vi "Database.GetAllStatus.vi"(8 "error in":errorcluster, 9 "Serial":string, 10 "Variant":string, 11 "Data in":T1) -> (0 "error out":errorcluster, 3 "Data out":T1)   [LabVIEW 2016]
uses:
  Database.Data.ctl
  Database.Data.Sets.ctl
  Handler/Database.Handler.Data.Status.ctl
  Database.Gui.ctl
  Database.Gui.SingleTestValue.ctl
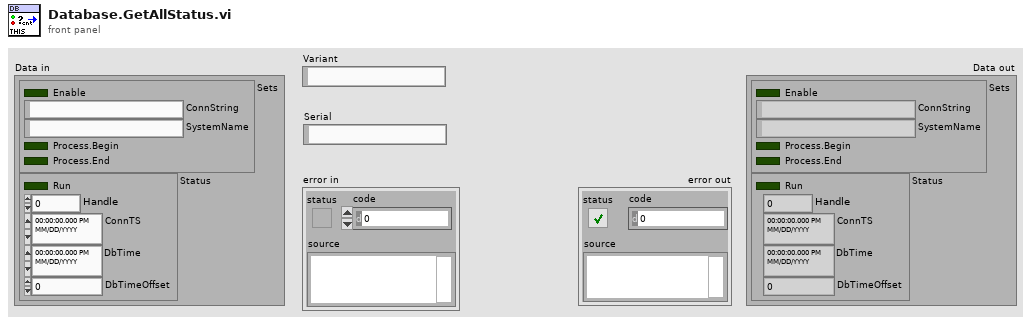
[diagram p1: front panel]
types:
  T1 = typedef "Database.Data.ctl" = cluster{"Sets":T2, "Status":T3}
  T2 = typedef "Database.Data.Sets.ctl" = cluster{"Enable":bool, "ConnString":string, "SystemName":string, "Process.Begin":bool, "Process.End":bool}
  T3 = typedef "Database.Handler.Data.Status.ctl" = cluster{"Run":bool, "Handle":i32, "ConnTS":timestamp, "DbTime":timestamp, "DbTimeOffset":dbl}
  T4 = typedef "Database.Gui.SingleTestValue.ctl" = cluster{"EV_name":string, "Value":dbl, "LimitL":dbl, "LimitH":dbl, "Status":u8}
  T5 = typedef "Database.Gui.ctl" = cluster{"Station":string, "ButtonEnabled":bool, "Values":T4[]}
  T6 = typedef "ProdaNG.Identification.ctl" = cluster{"processId":i32, "systemId":i32, "processStepId":i32, "wabcoPartId":i32}
  T7 = typedef "ProdaNG.Product.ctl" = cluster{"c_id":string, "wabcoPartId":i32, "serialNumber":string, "comment":string, "individual":i32, "crProcessStepId":i32, "mdProcessStepId":i32, "crTime":string, "mdTime":string}
  T8 = typedef "ProdaNG.TestStep.ctl" = cluster{"i_id":i32, "processStepId":i32, "testSequence":i32, "testOrder":i32, "mdReason":string, "mdUser":string, "mdTime":string, "description":string}
  T9 = typedef "ProdaNG.TestValue.ctl" = cluster{"i_id":i32, "testStepId":i32, "releaseId":i32, "unitId":i32, "contentId":string, "previewId":string, "maximum":dbl, "minimum":dbl, "valueText":string, "testValueSequence":i32, "history":i32, "mdReason":string, "mdUser":string, "mdTime":string, "description":string}
  T10 = typedef "ProdaNG.ProcessResult.ctl" = cluster{"c_id":string, "productId":string, "processId":i32, "statusId":i32, "startTime":string, "endTime":string}
  T11 = typedef "ProdaNG.ProcessStepResult.ctl" = cluster{"c_id":string, "processResultId":string, "processStepId":i32, "statusId":i32, "operatorId":i32, "startTime":string, "endTime":string}
  T12 = typedef "ProdaNG.TestStepResult.ctl" = cluster{"c_id":string, "processStepResultId":string, "testStepId":i32, "statusId":i32}
  T13 = typedef "ProdaNG.TestValueResult.ctl" = cluster{"c_id":string, "testStepResultId":string, "testValueId":i32, "result":dbl, "statusId":i32, "contentId":string}
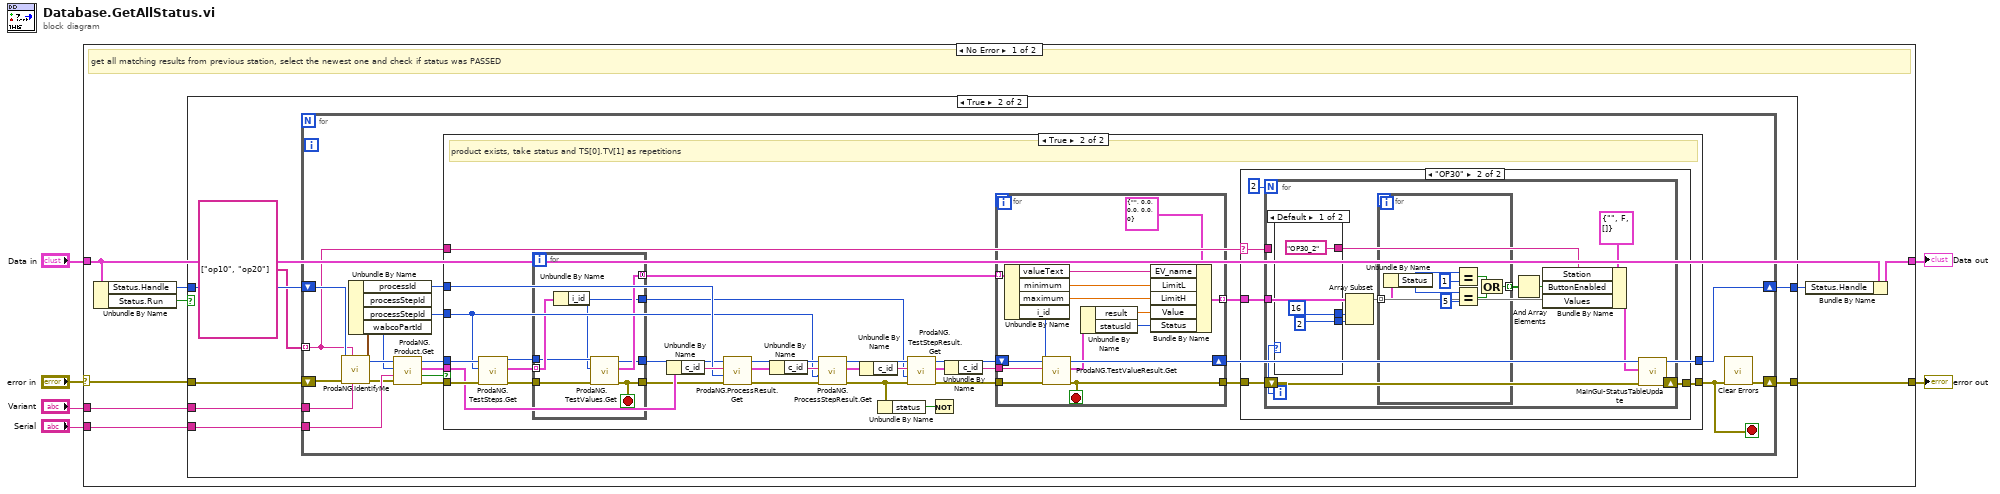
[diagram p0: block diagram]
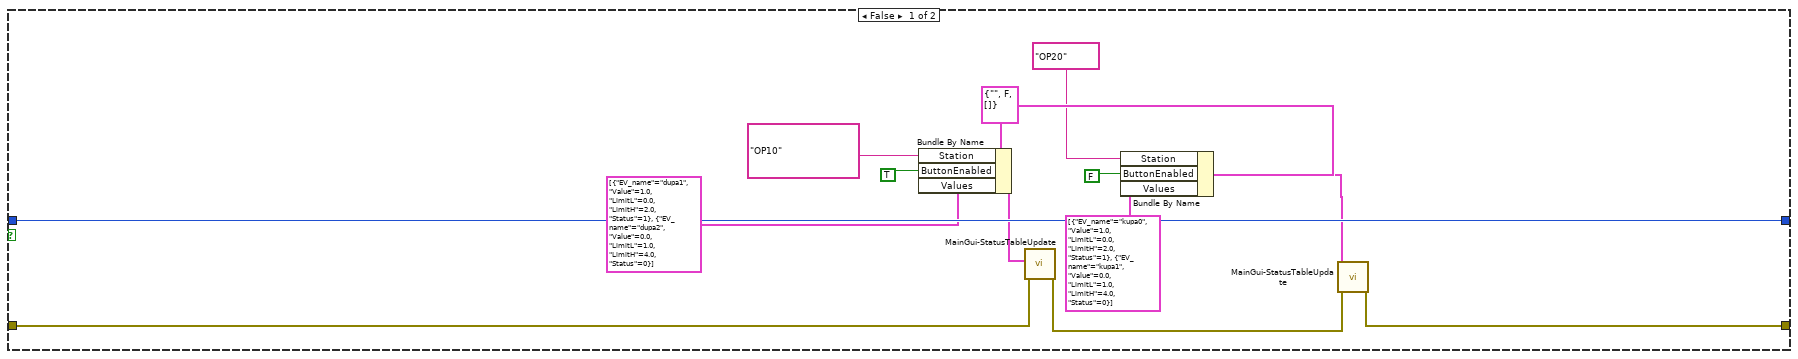
[diagram p2: hidden frame]
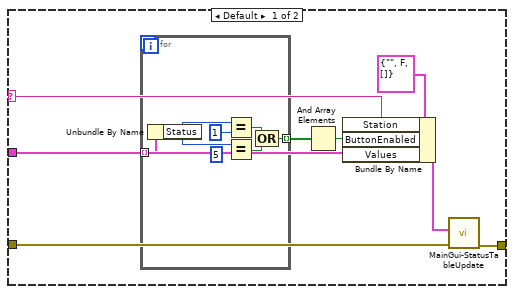
[diagram p4: hidden frame]
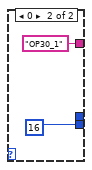
[diagram p5: hidden frame]
diagram:
  n1 = case shown="No Error" "error in" {
    selector: "error in" -> [w14 w154]
    tunnel: [w15 w154] -> w6
    tunnel: "Data in" -> [w12 w153]
    tunnel: [w11 w153] -> w3
    tunnel: "Serial" -> [w8 _]
    tunnel: "Variant" -> [w7 _]
    frame No Error {
      # "get all matching results from previous station, select the newest one and check if status was PASSED"
      n2 = Unbundle By Name(w12) -> ("Status.Handle"=w13:i32, "Status.Run"=w9:bool)
      n3 = case shown="True" w9 {
        tunnel: w14 -> [w26 w32]
        tunnel: [w21 w29] -> w15
        tunnel: w13 -> [w28 w34]
        tunnel: [w28 w35] -> w10
        tunnel: w8 -> [_ w33]
        tunnel: w7 -> [_ w30]
        frame False {
          w20 = T5 {"Station"="", "ButtonEnabled"=FALSE, "Values"=[]} ("TestValueResult")
          n4 = Bundle By Name(cluster=w20, "Station"="OP10", "ButtonEnabled"=TRUE, "Values"=T4[] [{"EV_name"="dupa1", "Value"=1.0, "LimitL"=0.0, "LimitH"=2.0, "Status"=1}, {"EV_name"="dupa2", "Value"=0.0, "LimitL"=1.0, "LimitH"=4.0, "Status"=0}]) -> (w27:T5)
          n5 = call "MainGui-StatusTableUpdate.vi"("error in (no error)"=w26, "TestValueResult"=w27) -> ("error out"=w22:errorcluster)  [unwired: 9 in]
          n6 = Bundle By Name(cluster=w20, "Station"="OP20", "ButtonEnabled"=FALSE, "Values"=T4[] [{"EV_name"="kupa0", "Value"=1.0, "LimitL"=0.0, "LimitH"=2.0, "Status"=1}, {"EV_name"="kupa1", "Value"=0.0, "LimitL"=1.0, "LimitH"=4.0, "Status"=0}]) -> (w17:T5)
          n7 = call "MainGui-StatusTableUpdate.vi"("error in (no error)"=w22, "TestValueResult"=w17) -> ("error out"=w21:errorcluster)  [unwired: 9 in]
        }
        frame True {
          n8 = for {
            tunnel: w33 -> [w47]
            shift-right: [w53] -> w29
            shift-left: w32 -> [w46]
            shift-right: [w48] -> w35
            shift-left: w34 -> [w45]
            tunnel: string[] ["op10", "op20"] -> [w38] mode=indexing
            tunnel: w30 -> [w37]
            stop <- w36 stop-if-true
            n9 = call "ProdaNG.IdentifyMe.vi"("wabcoNumber"=w37, "systemName"=w38, "error in"=w46, "dbHandleIn"=w45) -> ("error out"=w42:errorcluster, "Identification"=w43:T6, "dbHandle"=w44:i32)  [unwired: 5 in]
            n10 = Unbundle By Name(w43) -> ("processId"=w40:i32, "processStepId"=w39:i32, "wabcoPartId"=w41:i32)  [unwired: 1 out]
            n11 = call "ProdaNG.Product.Get.vi"("error in (no error)"=w42, "serialNumber"=w47, "wabcoPartId"=w41, "dbHandle"=w44) -> ("error out"=w51:errorcluster, "found"=w49:bool, "Product"=w50:T7, "dbHandle out"=w52:i32)  [unwired: 4 in]
            n12 = case shown="True" w49 {
              tunnel: w51 -> [w55 w70]
              tunnel: [w55 w59] -> w36
              tunnel: w52 -> [w54 w69]
              tunnel: w50 -> [_ w68]
              tunnel: [w54 w74] -> w48
              tunnel: w40 -> [_ w71]
              tunnel: w39 -> [_ w57]
              tunnel: w38 -> [_ w56]
              frame False {
                # "product missing"
              }
              frame True {
                # "product exists, take status and TS[0].TV[1] as repetitions"
                n13 = call "ProdaNG.TestSteps.Get.vi"("error in (no error)"=w70, "processStepId"=w57, "dbHandleIn"=w69) -> ("error out"=w65:errorcluster, "TestSteps"=w67:T8[], "dbHandle"=w66:i32)  [unwired: 6 in]
                n14 = for {
                  tunnel: w67 -> [w152] mode=indexing
                  tunnel: w66 -> [w149]
                  tunnel: w65 -> [w151]
                  tunnel: [w150] -> w62 mode=concatenating
                  tunnel: [w148] -> w64
                  tunnel: [w147] -> w63
                  tunnel: [w146] -> w58
                  stop <- w148 stop-if-true
                  n15 = Unbundle By Name(w152) -> ("i_id"=w146:i32)
                  n16 = call "ProdaNG.TestValues.Get.vi"("error in (no error)"=w151, "testStepId"=w146, "dbHandleIn"=w149) -> ("error out"=w148:errorcluster, "TestStepValues"=w150:T9[], "dbHandle"=w147:i32)  [unwired: 6 in]
                }
                n17 = Unbundle By Name(w68) -> ("c_id"=w82:string)
                n18 = call "ProdaNG.ProcessResult.Get.vi"("error in (no error)"=w64, "processId"=w71, "productId"=w82, "dbHandle"=w63) -> ("error out"=w84:errorcluster, "ProcessResult"=w86:T10, "dbHandle out"=w85:i32)  [unwired: 4 in, 1 out]
                n19 = Unbundle By Name(w86) -> ("c_id"=w83:string)
                n20 = call "ProdaNG.ProcessStepResult.Get.vi"("error in (no error)"=w84, "processStepId"=w57, "processResultId"=w83, "dbHandle"=w85) -> ("error out"=w73:errorcluster, "ProcessStepResult"=w79:T11, "dbHandle out"=w80:i32)  [unwired: 4 in, 1 out]
                n21 = Unbundle By Name(w79) -> ("c_id"=w78:string)
                n22 = Unbundle By Name(w73) -> ("status"=w72:bool)
                n23 = call "ProdaNG.TestStepResult.Get.vi"("error in (no error)"=w73, "testStepId"=w58, "processStepResulttId"=w78, "dbHandle"=w80) -> ("error out"=w76:errorcluster, "TestStepResult"=w81:T12, "dbHandle out"=w77:i32)  [unwired: 4 in, 1 out]
                n24 = Not(x=w72) -> ()  [unwired: 1 out]
                n25 = Unbundle By Name(w81) -> ("c_id"=w75:string)
                n26 = for {
                  tunnel: w75 -> [w143]
                  shift-right: [w142] -> w74
                  shift-left: w77 -> [w145]
                  tunnel: w76 -> [w144]
                  tunnel: [w141] -> w60
                  tunnel: w62 -> [w140] mode=indexing
                  tunnel: [w131] -> w61 mode=indexing
                  stop <- w141 stop-if-true
                  n27 = Unbundle By Name(w140) -> ("valueText"=w136:string, "minimum"=w135:dbl, "maximum"=w134:dbl, "i_id"=w139:i32)
                  n28 = call "ProdaNG.TestValueResult.Get.vi"("error in (no error)"=w144, "testValueId"=w139, "testStepResultId"=w143, "dbHandle"=w145) -> ("error out"=w141:errorcluster, "TestValueResult"=w138:T13, "dbHandle"=w142:i32)  [unwired: 5 in]
                  n29 = Unbundle By Name(w138) -> ("result"=w133:dbl, "statusId"=w132:i32)
                  n30 = Bundle By Name(cluster=T4 {"EV_name"="", "Value"=0.0, "LimitL"=0.0, "LimitH"=0.0, "Status"=0} ("Cluster"), "EV_name"=w136, "LimitL"=w135, "LimitH"=w134, "Value"=w133, "Status"=w132) -> (w131:T4)
                }
                n31 = case shown="\"OP30\"" w56 {
                  selector: w56 -> [w87 w104]
                  tunnel: w61 -> [w91 w103]
                  tunnel: w60 -> [w90 w106]
                  tunnel: [w89 w105] -> w59
                  frame Default {
                    n32 = for {
                      tunnel: w91 -> [w95] mode=indexing
                      tunnel: [w96] -> w94 mode=indexing
                      n33 = Unbundle By Name(w95) -> ("Status"=w101:u8)
                      n34 = Equal?(x=w101, y=u8 1) -> (x = y?=w98:bool)
                      n35 = Equal?(x=w101, y=u8 5) -> (x = y?=w97:bool)
                      n36 = Compound Arithmetic op=OR(w98, w97) -> (w96:bool)
                    }
                    n37 = And Array Elements(Boolean array=w94) -> (logical AND=w92:bool)
                    n38 = Bundle By Name(cluster=T5 {"Station"="", "ButtonEnabled"=FALSE, "Values"=[]} ("TestValueResult"), "Station"=w87, "ButtonEnabled"=w92, "Values"=w91) -> (w88:T5)
                    n39 = call "MainGui-StatusTableUpdate.vi"("error in (no error)"=w90, "TestValueResult"=w88) -> ("error out"=w89:errorcluster)  [unwired: 9 in]
                  }
                  frame "OP30" {
                    n40 = for {
                      N: 2 -> [_]
                      tunnel: w104 -> [_]
                      tunnel: w103 -> [w112]
                      shift-right: [w114] -> w105
                      shift-left: w106 -> [w115]
                      i -> [w110]
                      n41 = case shown="Default" w110 {
                        tunnel: [2 16] -> w109
                        tunnel: [16 _] -> w108
                        tunnel: ["OP30_2" "OP30_1"] -> w107
                        frame Default {
                        }
                        frame 0 {
                        }
                      }
                      n42 = Array Subset(array=w112, index=w108, length=w109) -> (w111:T4[])
                      n43 = for {
                        tunnel: w111 -> [w124] mode=indexing
                        tunnel: [w125] -> w118 mode=indexing
                        n44 = Unbundle By Name(w124) -> ("Status"=w130:u8)
                        n45 = Equal?(x=w130, y=u8 1) -> (x = y?=w127:bool)
                        n46 = Equal?(x=w130, y=u8 5) -> (x = y?=w126:bool)
                        n47 = Compound Arithmetic op=OR(w127, w126) -> (w125:bool)
                      }
                      n48 = And Array Elements(Boolean array=w118) -> (logical AND=w116:bool)
                      n49 = Bundle By Name(cluster=T5 {"Station"="", "ButtonEnabled"=FALSE, "Values"=[]} ("TestValueResult"), "Station"=w107, "ButtonEnabled"=w116, "Values"=w111) -> (w113:T5)
                      n50 = call "MainGui-StatusTableUpdate.vi"("error in (no error)"=w115, "TestValueResult"=w113) -> ("error out"=w114:errorcluster)  [unwired: 9 in]
                    }
                  }
                }
              }
            }
            n51 = call <vilib>:"Clear Errors.vi"("error in (no error)"=w36) -> ("error out"=w53:errorcluster)  [unwired: 5 in, 1 out]
          }
        }
      }
      n52 = Bundle By Name(cluster=w12, "Status.Handle"=w10) -> (w11:T1)
    }
    frame Error {
    }
  }
  "error out" <- w6
  "Data out" <- w3
